vi "CheckTure.vi"(0 "Bool引用":refnum<vi>, 5 "Array引用":refnum<vi>, 7 "索引":i32, 9 "长度":i32, 11 "错误输入（无错误）":errorcluster) -> (15 "错误输出":errorcluster)   [LabVIEW 2011]
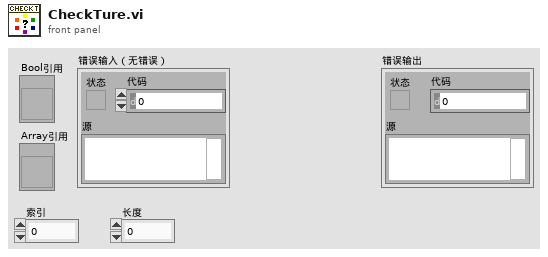
[diagram p1: front panel]
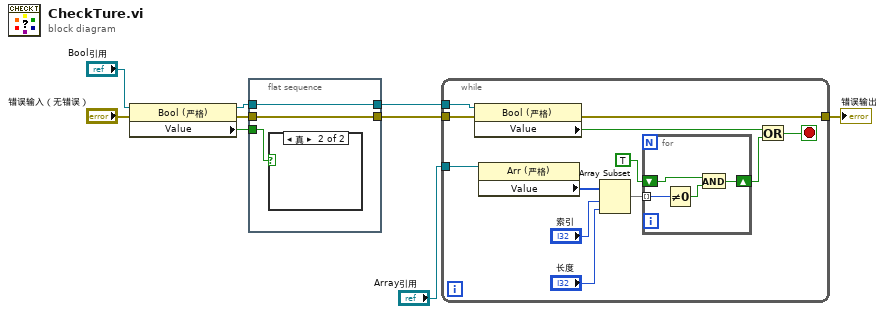
[diagram p0: block diagram]
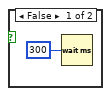
[diagram p2: hidden frame]
diagram:
  n1 = property class="Bool (严格)"(reference="Bool引用", error in="错误输入（无错误）") -> (reference out=w5:refnum<vi>, error out=w7:errorcluster, "Value"=w6:bool)
  n2 = flat-sequence {
    tunnel: [w12] -> w2
    tunnel: w7 -> [w12]
    tunnel: w6 -> [w10]
    tunnel: [w11] -> w3
    tunnel: w5 -> [w11]
    frame #0 {
      n3 = case shown="真" w10 {
        frame False {
          n4 = Wait (ms)(milliseconds to wait=u32 300 ("等待时间（毫秒）")) -> ()  [unwired: 1 out]
        }
        frame True {
        }
      }
    }
  }
  n5 = while {
    tunnel: "Array引用" -> [w21]
    tunnel: w3 -> [w25]
    tunnel: w2 -> [w24]
    tunnel: [w17] -> w1
    stop <- w22 stop-if-true
    n6 = property class="Bool (严格)"(reference=w25, error in=w24) -> (error out=w17:errorcluster, "Value"=w23:bool)  [unwired: 1 out]
    n7 = property class="Arr (严格)"(reference=w21) -> ("Value"=w20:i32[])  [unwired: 1 in, 2 out]
    n8 = Array Subset(array=w20, index="索引", length="长度") -> (w16:i32[])
    n9 = for {
      tunnel: w16 -> [w28] mode=indexing
      shift-right: [w26] -> w14
      shift-left: TRUE -> [w29]
      n10 = Not Equal To 0?(x=w28) -> (x != 0?=w27:bool)
      n11 = And(x=w29, y=w27) -> (x .and. y?=w26:bool)
    }
    n12 = Or(x=w23, y=w14) -> (x .or. y?=w22:bool)
  }
  "错误输出" <- w1
